vi "Wait if Occupied.vi"(8 "View":i32[](array[numeric]) caption="View (Team Index, -1: empty)", 9 "Direction In":T1, 11 "Action In":T2) -> (1 "Direction Out":T1, 3 "Action Out":T2)   [LabVIEW 2015, in "Common.lvlib"]
uses:
  Type Defs/Action Enum.ctl
  Type Defs/Direction Enum.ctl
  Common.lvlib
  Type Defs/SB Type Defs.lvlib
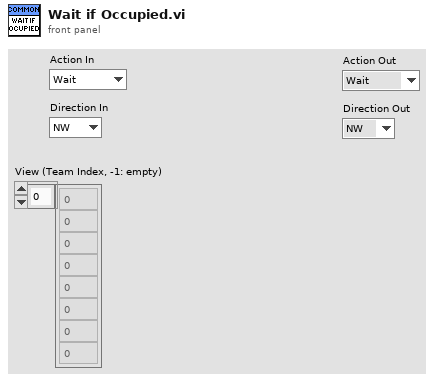
[diagram p1: front panel]
types:
  T1 = typedef "SB Type Defs.lvlib/Direction Enum.ctl" = enum16{"NW", "N", "NE", "E", "SE", "S", "SW", "W"}
  T2 = typedef "SB Type Defs.lvlib/Action Enum.ctl" = enum16{"Wait", "Move", "Attack", "Replicate"}
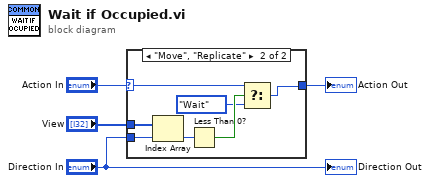
[diagram p0: block diagram]
diagram:
  n1 = case shown="\"Move\", \"Replicate\"" "Action In" {
    selector: "Action In" -> [w5 w10]
    tunnel: [w5 w8] -> w3
    tunnel: "Direction In" -> [_ w7]
    tunnel: "View" -> [_ w12]
    frame "Wait", "Attack" {
    }
    frame "Move", "Replicate" {
      n2 = Index Array(array=w12, index=w7) -> (element=w11:i32)
      n3 = Less Than 0?(x=w11) -> (x < 0?=w9:bool)
      n4 = Select(t=w10, s=w9, f=Action_Enum."Wait") -> (s? t:f=w8:T2)
    }
  }
  "Action Out" <- w3
  "Direction Out" <- "Direction In"
